vi "REG - 2DSortData.vi"(7 "Index":cluster{"X":i32, "Y":i32}, 8 "error in":errorcluster, 10 "Y":dbl[](array[numeric]), 11 "X":dbl[][](array[numeric])) -> (0 "error out":errorcluster, 3 "Array":cluster{"Array":dbl[], "Array":dbl[]}[](array[cluster]))   [LabVIEW 2020]
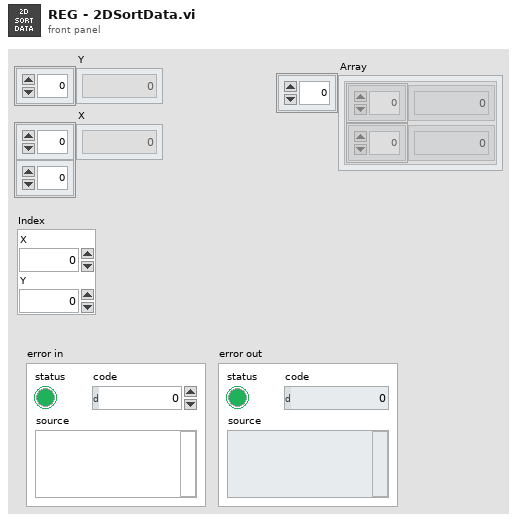
[diagram p1: front panel]
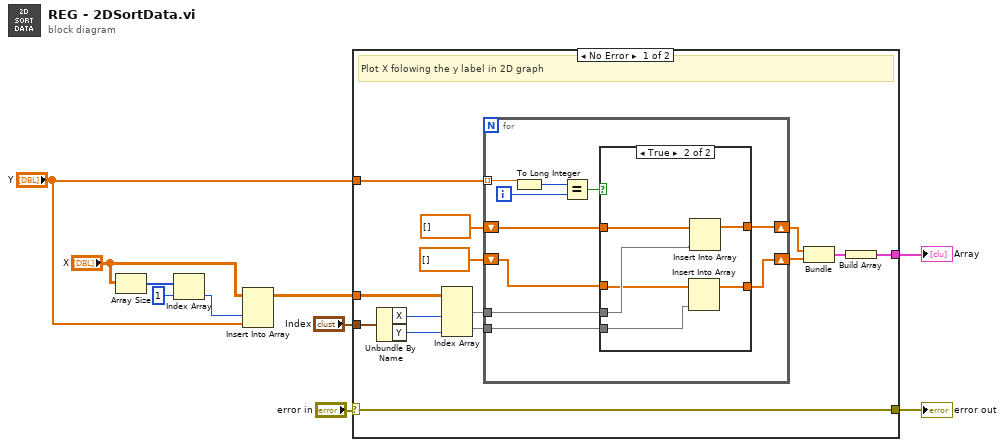
[diagram p0: block diagram]
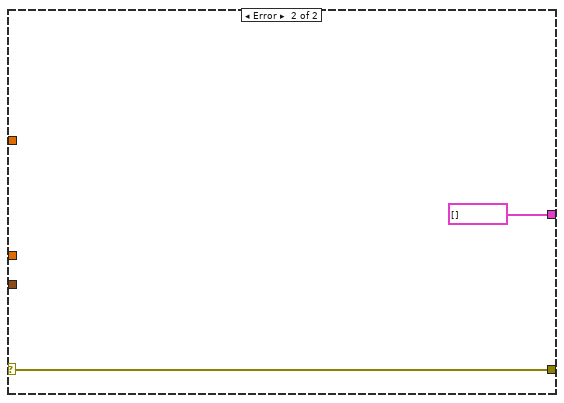
[diagram p3: hidden frame]
diagram:
  n1 = Array Size(array="X") -> (size(s)=w3:i32[])
  n2 = Index Array(array=w3, index=1) -> (element=w1:i32)
  n3 = Insert Into Array(array="X", index (col)=w1, new element="Y") -> (w6:dbl[][])  [unwired: 1 in]
  n4 = case shown="No Error" "error in" {
    selector: "error in" -> [w22 w44]
    tunnel: w6 -> [w21 _]
    tunnel: "Y" -> [w17 _]
    tunnel: [w22 w44] -> w7
    tunnel: [w13 cluster{dbl[], dbl[]}[] []] -> w9
    tunnel: "Index" -> [w20 _]
    frame No Error {
      # "Plot X folowing the y label in 2D graph"
      n5 = Unbundle By Name(w20) -> ("X"=w19:i32, "Y"=w18:i32)
      n6 = Index Array(array=w21, index (col) #1=w19, index (col) #2=w18) -> (element #1=w24:dbl[], element #2=w23:dbl[])  [unwired: 2 in]
      n7 = for {
        tunnel: w24 -> [w34]
        tunnel: w23 -> [w33]
        tunnel: w17 -> [w32] mode=indexing
        shift-right: [w30] -> w16
        shift-left: dbl[] [] -> [w26]
        shift-right: [w25] -> w15
        shift-left: dbl[] [] -> [w27]
        i -> [w31]
        n8 = To Long Integer(number=w32) -> (32bit integer=w29:i32)
        n9 = Equal?(x=w29, y=w31) -> (x = y?=w28:bool)
        n10 = case shown="True" w28 {
          tunnel: w34 -> [_ w41]
          tunnel: w33 -> [_ w37]
          tunnel: [w35 w39] -> w25
          tunnel: [w36 w40] -> w30
          tunnel: w26 -> [w36 w42]
          tunnel: w27 -> [w35 w38]
          frame False {
          }
          frame True {
            n11 = Insert Into Array(array=w38, new element=w37) -> (w39:dbl[])  [unwired: 1 in]
            n12 = Insert Into Array(array=w42, new element=w41) -> (w40:dbl[])  [unwired: 1 in]
          }
        }
      }
      n13 = Bundle(w16, w15) -> (w14:cluster{dbl[], dbl[]})  [unwired: 1 in]
      n14 = Build Array(w14) -> (w13:cluster{dbl[], dbl[]}[])
    }
    frame Error {
    }
  }
  "Array" <- w9
  "error out" <- w7
